vi "Calculate R and G 2.vi"(9 "Electrodes":T1(array[cluster]), 10 "Excitation":dbl[](array[numeric]), 11 "Data (V or A)":dbl[](array[numeric])) -> (0 "G_4T (S)":dbl[](array[numeric]), 1 "R_4T (Ohms)":dbl[](array[numeric]), 2 "G_2T (S)":dbl[](array[numeric]), 3 "R_2T (Ohms)":dbl[](array[numeric]))   [LabVIEW 2019, in "Transport.lvclass"]
uses:
  Transport.lvclass
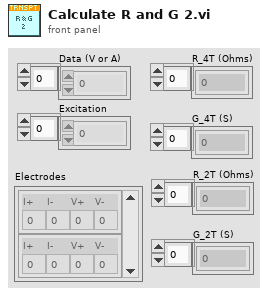
[diagram p1: front panel]
types:
  T1 = cluster{"I+":i32, "I-":i32, "V+":i32, "V-":i32}[]
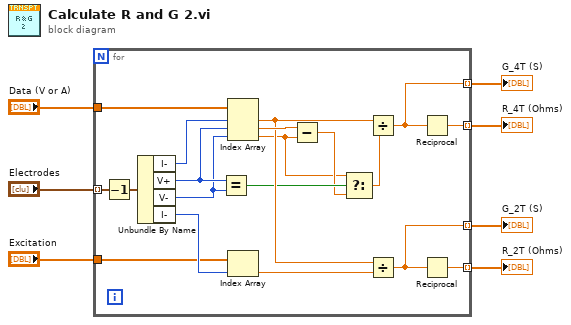
[diagram p0: block diagram]
diagram:
  n1 = for {
    tunnel: "Data (V or A)" -> [w26]
    tunnel: [w23] -> w5 mode=indexing
    tunnel: [w24] -> w4 mode=indexing
    tunnel: "Electrodes" -> [w22] mode=indexing
    tunnel: [w17] -> w2 mode=indexing
    tunnel: [w18] -> w3 mode=indexing
    tunnel: "Excitation" -> [w15]
    n2 = Decrement(x=w22) -> (x-1=w21:cluster{"I+":i32, "I-":i32, "V+":i32, "V-":i32})
    n3 = Unbundle By Name(w21) -> ("I-"=w20:i32, "V+"=w12:i32, "V-"=w11:i32, "I-"=w16:i32)
    n4 = Equal?(x=w12, y=w11) -> (x = y?=w13:bool)
    n5 = Index Array(array=w26, index #1=w20, index #2=w12, index #3=w11) -> (element #1=w19:dbl, element #2=w25:dbl, element #3=w8:dbl)
    n6 = Index Array(array=w15, index=w16) -> (element=w14:dbl)
    n7 = Subtract(x=w25, y=w8) -> (x-y=w9:dbl)
    n8 = Select(t=w8, s=w13, f=w9) -> (s? t:f=w10:dbl)
    n9 = Divide(x=w19, y=w10) -> (x/y=w23:dbl)
    n10 = Divide(x=w19, y=w14) -> (x/y=w17:dbl)
    n11 = Reciprocal(x=w23) -> (1/x=w24:dbl)
    n12 = Reciprocal(x=w17) -> (1/x=w18:dbl)
  }
  "G_4T (S)" <- w5
  "R_4T (Ohms)" <- w4
  "G_2T (S)" <- w2
  "R_2T (Ohms)" <- w3
